vi "setOutputLoad.vi"(8 "error in (no error)":errorcluster, 10 "Phase":dbl(ring) items=["50"=50.0, "75"=75.0, "HighZ"=0.0], 11 "VISA resource name":refnum<visa-resource-name>) -> (0 "error out":errorcluster, 3 "VISA resource name out":refnum<visa-resource-name>)   [LabVIEW 2023, in "Keysight-33500B.lvlib"]
doc: "<b>Author:</b> Wolfgang\n<b>Description:</b>\nSets the starting phase angle for the burst. in degree"
uses:
  Keysight-33500B.lvlib
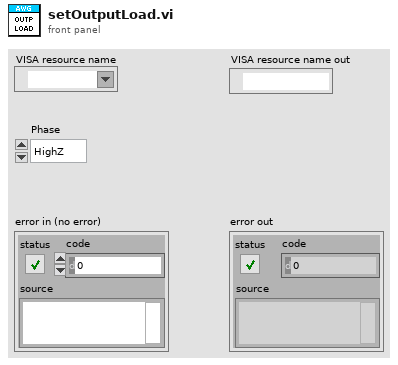
[diagram p1: front panel]
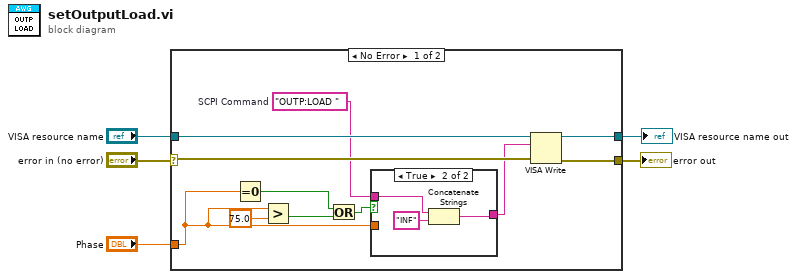
[diagram p0: block diagram]
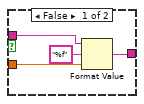
[diagram p2: hidden frame]
diagram:
  n1 = case shown="No Error" "error in (no error)" {
    selector: "error in (no error)" -> [w13 w25]
    tunnel: [w15 w24] -> w5
    tunnel: [w16 w25] -> w3
    tunnel: "VISA resource name" -> [w14 w24]
    tunnel: "Phase" -> [w9 _]
    frame No Error {
      w12 = "OUTP:LOAD "  # SCPI Command
      n2 = Equal To 0?(x=w9) -> (x = 0?=w10:bool)
      n3 = Greater?(x=w9, y=75.0) -> (0:w6:bool)
      n4 = Or(x=w10, y=w6) -> (x .or. y?=w7:bool)
      n5 = case shown="True" w7 {
        tunnel: w12 -> [w20 w23]
        tunnel: [w19 w22] -> w11
        tunnel: w9 -> [w17 _]
        frame False {
          n6 = Format Value(string ("")=w20, format string="%f", value (0)=w17) -> (output string=w19:string)
        }
        frame True {
          n7 = Concatenate Strings(w23, "INF" ("string")) -> (w22:string)
        }
      }
      n8 = VISA Write(VISA resource name=w14, write buffer=w11, error in (no error)=w13) -> (VISA resource name out=w15:refnum<visa-resource-name>, error out=w16:errorcluster)  [unwired: 1 out]
    }
    frame Error {
    }
  }
  "VISA resource name out" <- w5
  "error out" <- w3
